vi "Get PhXP Parameters.vi"(8 "Error In":errorcluster) -> (0 "Error Out":errorcluster, 1 "tau*":dbl[unit]=1.9894367886486918e-09 format="%#_5g", 2 "f0":dbl[unit]=80000000.0 format="%#_5g", 3 "Phasor Explorer Parameters":T1={"Display Parameters"={"# Points"=0, "Ramp Type"=enum."Linear", "Type of Series"=enum."1-Exp Decays", "Min tau"=0.0, "Max tau"=0.0, "Include 0"=FALSE, "Include Infinity"=FALSE}, "Phasor Parameters"={"Harmonic frequency"=0.0, "Use f* = 1/D Frequency"=FALSE, "Calibrated Phasor"=FALSE, "Calibration Lifetime"=0.0, "Phasor Calculation"=enum."Direct Sum", "SEPL Type"=enum."UC", "# Gates"=1.0, "Square Gate Width"=1e-09, "Show Ticks"=FALSE}, "Decay & IRF Parameters"={"Lifetime"=0.0, "IRF Offset"=0.0, "Laser Period"=0.0, "Normalized Decays"=FALSE, "IRF Model"=enum."Dirac", "IRF Parameter 1"=0.0}, "Gate Parameters"={"First Gate Start"=0.0, "Use Gate Center"=FALSE, "Gate Width"=0.0, "Gate Step"=0.0, "# Gates"=0.0, "Gate Type"=enum."Square", "Edge Width"=0.0, "Top Slope"=0.0, "Reversed Sawtooth?"=FALSE, "Analytical Computation"=FALSE, "Tolerance"=1.0, "Integration"=enum."Item 0", "# Steps"=1.0, "Type of User-defined Function"=enum."Gate"}, "Detector Parameters"={"Frames/Image"=0, "Gates/Frame"=0, "Bits/Frame"=0, "Multiplicity"=0, "Incident Signal"=0.0}} {"Detector Parameters"."Frames/Image" min=1; "Detector Parameters"."Multiplicity" min=0; "Detector Parameters"."Bits/Frame" min=1; "Detector Parameters"."Gates/Frame" min=1; "Gate Parameters"."# Steps" min=0.0; "Gate Parameters"."Tolerance" min=0.0; "Gate Parameters"."Top Slope" min=0.0; "Gate Parameters"."Edge Width" min=0.0; "Gate Parameters"."Gate Step" min=0.0; "Gate Parameters"."# Gates" min=0.0 step=1.0; "Gate Parameters"."Gate Width" min=0.0; "Decay & IRF Parameters"."Lifetime" min=0.0; "Decay & IRF Parameters"."Laser Period" min=0.0; "Phasor Parameters"."Square Gate Width" min=0.0; "Phasor Parameters"."# Gates" min=0.0; "Phasor Parameters"."Calibration Lifetime" min=0.0; "Phasor Parameters"."Harmonic frequency" min=0.0; "Display Parameters"."Min tau" min=0.0; "Display Parameters"."Max tau" min=0.0; "Display Parameters"."# Points" min=1 step=1})   [LabVIEW 2019]
uses:
  Pseudo Phasor Parameters.ctl
  Phasor Explorer Display Parameters.ctl
  Type of Series.ctl
  Phasor Explorer Phasor Parameters.ctl
  Phasor Calculation Type.ctl
  Phasor Type.ctl
  Phasor Explorer Decay Parameters.ctl
  IRF Model.ctl
  Phasor Explorer Gate Parameters.ctl
  Gate Type.ctl
  Phasor Explorer Detector Parameters.ctl
  Phasor Explorer Settings List.ctl
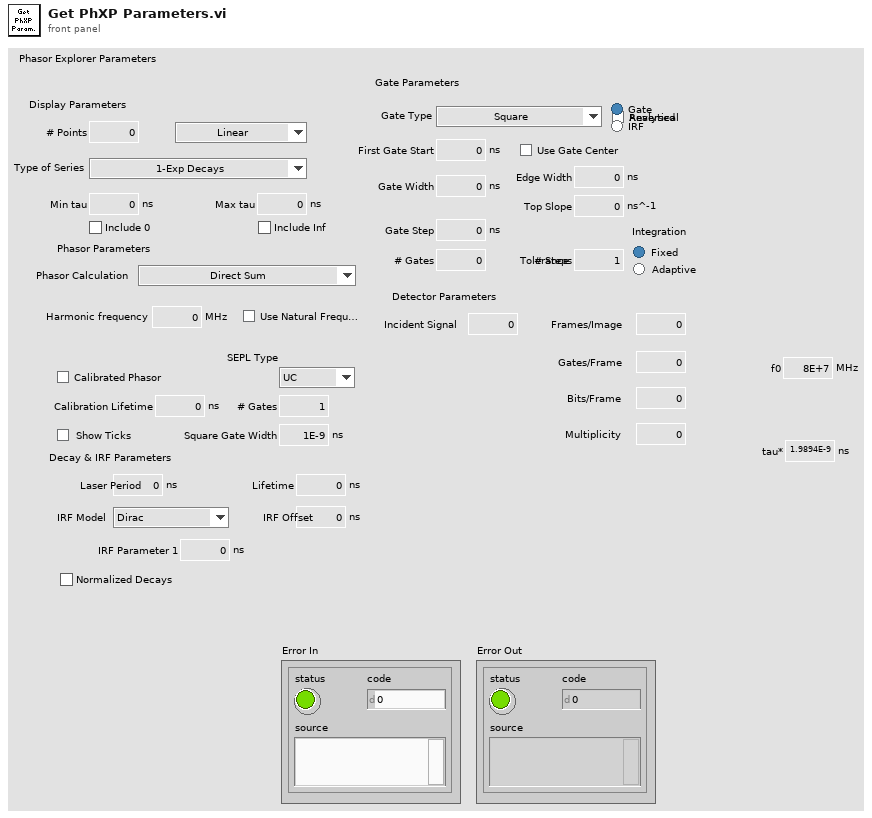
[diagram p1: front panel]
types:
  T1 = typedef "Pseudo Phasor Parameters.ctl" = cluster{"Display Parameters":T2, "Phasor Parameters":T4, "Decay & IRF Parameters":T7, "Gate Parameters":T9, "Detector Parameters":T11}
  T2 = typedef "Phasor Explorer Display Parameters.ctl" = cluster{"# Points":i32, "Ramp Type":enum16{"Linear", "Logarithmic"}, "Type of Series":T3, "Min tau":dbl[unit], "Max tau":dbl[unit], "Include 0":bool, "Include Infinity":bool}
  T3 = typedef "Type of Series.ctl" = enum16{"1-Exp Decays", "Linear Combination of 1-Exp"}
  T4 = typedef "Phasor Explorer Phasor Parameters.ctl" = cluster{"Harmonic frequency":dbl[unit], "Use f* = 1/D Frequency":bool, "Calibrated Phasor":bool, "Calibration Lifetime":dbl[unit], "Phasor Calculation":T5, "SEPL Type":T6, "# Gates":dbl, "Square Gate Width":dbl[unit], "Show Ticks":bool}
  T5 = typedef "Phasor Calculation Type.ctl" = enum16{"Direct Sum", "Analytical Formula"}
  T6 = typedef "Phasor Type.ctl" = enum16{"UC", "L_N", "L_N[W]"}
  T7 = typedef "Phasor Explorer Decay Parameters.ctl" = cluster{"Lifetime":dbl[unit], "IRF Offset":dbl[unit], "Laser Period":dbl[unit], "Normalized Decays":bool, "IRF Model":T8, "IRF Parameter 1":dbl[unit]}
  T8 = typedef "IRF Model.ctl" = enum16{"Dirac", "Exponential"}
  T9 = typedef "Phasor Explorer Gate Parameters.ctl" = cluster{"First Gate Start":dbl[unit], "Use Gate Center":bool, "Gate Width":dbl[unit], "Gate Step":dbl[unit], "# Gates":dbl, "Gate Type":T10, "Edge Width":dbl[unit], "Top Slope":dbl[unit], "Reversed Sawtooth?":bool, "Analytical Computation":bool, "Tolerance":dbl, "Integration":enum32{"Item 0", "Item 1"}, "# Steps":dbl, "Type of User-defined Function":enum32{"Gate", "IRF"}}
  T10 = typedef "Gate Type.ctl" = enum16{"Square", "Finite Edge Square", "Finite Edge, Tilted Top Square", "Triangle", "Sawtooth", "User-defined"}
  T11 = typedef "Phasor Explorer Detector Parameters.ctl" = cluster{"Frames/Image":i32, "Gates/Frame":i32, "Bits/Frame":i32, "Multiplicity":i32, "Incident Signal":dbl}
  T12 = typedef "Phasor Explorer Settings List.ctl" = enum16{"Phasor Explorer Display Parameters", "Phasor Explorer Phasor Parameters", "Phasor Explorer Decay & IRF Parameters", "Phasor Explorer Gate Parameters", "Phasor Explorer Detector Parameters", "f*", "tau*"}
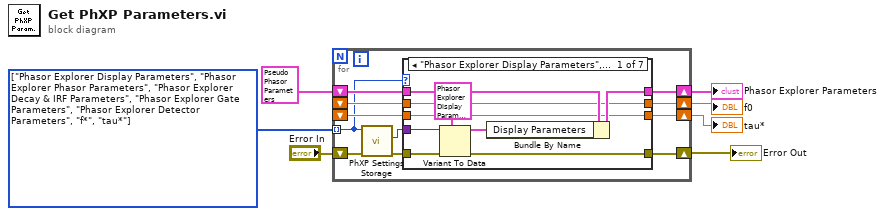
[diagram p0: block diagram]
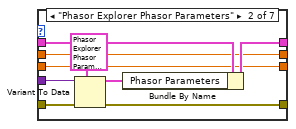
[diagram p2: hidden frame]
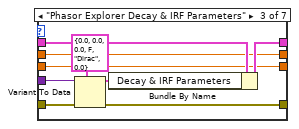
[diagram p3: hidden frame]
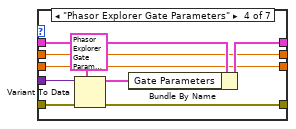
[diagram p4: hidden frame]
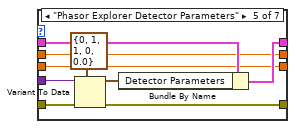
[diagram p5: hidden frame]
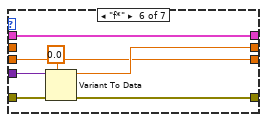
[diagram p6: hidden frame]
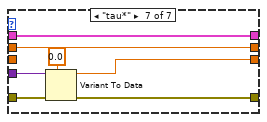
[diagram p7: hidden frame]
diagram:
  w5 = T12[] [enum."Phasor Explorer Display Parameters", enum."Phasor Explorer Phasor Parameters", enum."Phasor Explorer Decay & IRF Parameters", enum."Phasor Explorer Gate Parameters", enum."Phasor Explorer Detector Parameters", enum."f*", enum."tau*"] items=["Phasor Explorer Display Parameters", "Phasor Explorer Phasor Parameters", "Phasor Explorer Decay & IRF Parameters", "Phasor Explorer Gate Parameters", "Phasor Explorer Detector Parameters", "f*", "tau*"] ("Settings List")
  n1 = for {
    tunnel: w5 -> [w8] mode=indexing
    shift-right: [w17] -> w7
    shift-left: T1 {"Display Parameters"={"# Points"=0, "Ramp Type"=enum."Linear", "Type of Series"=enum."1-Exp Decays", "Min tau"=0.0, "Max tau"=0.0, "Include 0"=FALSE, "Include Infinity"=FALSE}, "Phasor Parameters"={"Harmonic frequency"=0.0, "Use f* = 1/D Frequency"=FALSE, "Calibrated Phasor"=FALSE, "Calibration Lifetime"=1e-09, "Phasor Calculation"=enum."Direct Sum", "SEPL Type"=enum."UC", "# Gates"=1.0, "Square Gate Width"=1e-09, "Show Ticks"=FALSE}, "Decay & IRF Parameters"={"Lifetime"=0.0, "IRF Offset"=0.0, "Laser Period"=0.0, "Normalized Decays"=FALSE, "IRF Model"=enum."Dirac", "IRF Parameter 1"=0.0}, "Gate Parameters"={"First Gate Start"=0.0, "Use Gate Center"=FALSE, "Gate Width"=0.0, "Gate Step"=0.0, "# Gates"=0.0, "Gate Type"=enum."Square", "Edge Width"=0.0, "Top Slope"=0.0, "Reversed Sawtooth?"=FALSE, "Analytical Computation"=FALSE, "Tolerance"=1.0, "Integration"=enum."Item 0", "# Steps"=1.0, "Type of User-defined Function"=enum."Gate"}, "Detector Parameters"={"Frames/Image"=0, "Gates/Frame"=0, "Bits/Frame"=0, "Multiplicity"=0, "Incident Signal"=0.0}} ("Phasor Explorer Parameters") -> [w18]
    shift-right: [w13] -> w3
    shift-left: "Error In" -> [w14]
    shift-right: [w12] -> w2
    shift-left: _ -> [w11]
    shift-right: [w10] -> w1
    shift-left: _ -> [w9]
    n2 = call "PhXP Settings Storage.vi"("Error In"=w14, "Settings List"=w8) -> ("Error Out"=w16:errorcluster, "Variant Data out"=w15:variant)  [unwired: 8 in]
    n3 = case shown="\"Phasor Explorer Display Parameters\", Default" w8 {
      tunnel: w18 -> [w27 w36 w45 w54 w63 w67 w74]
      tunnel: [w26 w35 w44 w53 w62 w67 w74] -> w17
      tunnel: w16 -> [w25 w34 w43 w52 w61 w70 w77]
      tunnel: w15 -> [w24 w33 w42 w51 w60 w69 w76]
      tunnel: [w21 w30 w39 w48 w57 w68 w75] -> w13
      tunnel: [w20 w29 w38 w47 w56 w65 w71] -> w12
      tunnel: w11 -> [w20 w29 w38 w47 w56 _ w71]
      tunnel: [w19 w28 w37 w46 w55 w64 w72] -> w10
      tunnel: w9 -> [w19 w28 w37 w46 w55 w64 _]
      frame "Phasor Explorer Display Parameters", Default {
        n4 = Variant To Data(error in=w25, type=T2 {"# Points"=1, "Ramp Type"=enum."Linear", "Type of Series"=enum."1-Exp Decays", "Min tau"=0.0, "Max tau"=0.0, "Include 0"=FALSE, "Include Infinity"=FALSE} ("Display Parameters"), Variant=w24) -> (data=w23:T2, error out=w21:errorcluster)
        n5 = Bundle By Name(cluster=w27, "Display Parameters"=w23) -> (w26:T1)
      }
      frame "Phasor Explorer Phasor Parameters" {
        n6 = Variant To Data(error in=w34, type=T4 {"Harmonic frequency"=0.0, "Use f* = 1/D Frequency"=FALSE, "Calibrated Phasor"=FALSE, "Calibration Lifetime"=1e-09, "Phasor Calculation"=enum."Direct Sum", "SEPL Type"=enum."UC", "# Gates"=1.0, "Square Gate Width"=1e-09, "Show Ticks"=FALSE} ("Phasor Parameters"), Variant=w33) -> (data=w32:T4, error out=w30:errorcluster)
        n7 = Bundle By Name(cluster=w36, "Phasor Parameters"=w32) -> (w35:T1)
      }
      frame "Phasor Explorer Decay & IRF Parameters" {
        n8 = Variant To Data(error in=w43, type=T7 {"Lifetime"=0.0, "IRF Offset"=0.0, "Laser Period"=0.0, "Normalized Decays"=FALSE, "IRF Model"=enum."Dirac", "IRF Parameter 1"=0.0} ("Decay Parameters"), Variant=w42) -> (data=w41:T7, error out=w39:errorcluster)
        n9 = Bundle By Name(cluster=w45, "Decay & IRF Parameters"=w41) -> (w44:T1)
      }
      frame "Phasor Explorer Gate Parameters" {
        n10 = Variant To Data(error in=w52, type=T9 {"First Gate Start"=0.0, "Use Gate Center"=FALSE, "Gate Width"=0.0, "Gate Step"=0.0, "# Gates"=1.0, "Gate Type"=enum."Square", "Edge Width"=0.0, "Top Slope"=0.0, "Reversed Sawtooth?"=FALSE, "Analytical Computation"=FALSE, "Tolerance"=1.0, "Integration"=enum."Item 0", "# Steps"=1.0, "Type of User-defined Function"=enum."Gate"} ("Gate Parameters"), Variant=w51) -> (data=w50:T9, error out=w48:errorcluster)
        n11 = Bundle By Name(cluster=w54, "Gate Parameters"=w50) -> (w53:T1)
      }
      frame "Phasor Explorer Detector Parameters" {
        n12 = Variant To Data(error in=w61, type=T11 {"Frames/Image"=0, "Gates/Frame"=1, "Bits/Frame"=1, "Multiplicity"=0, "Incident Signal"=0.0} ("Detector Parameters"), Variant=w60) -> (data=w59:T11, error out=w57:errorcluster)
        n13 = Bundle By Name(cluster=w63, "Detector Parameters"=w59) -> (w62:T1)
      }
      frame "f*" {
        n14 = Variant To Data(error in=w70, type=dbl[unit] 0.0 ("f0"), Variant=w69) -> (data=w65:dbl[unit], error out=w68:errorcluster)
      }
      frame "tau*" {
        n15 = Variant To Data(error in=w77, type=dbl[unit] 0.0 ("tau*"), Variant=w76) -> (data=w72:dbl[unit], error out=w75:errorcluster)
      }
    }
  }
  "Phasor Explorer Parameters" <- w7
  "Error Out" <- w3
  "tau*" <- w1
  "f0" <- w2
